vi "Gen - Remove Empty String Array.vi"(11 "Data Array":string[](array[string])) -> (3 "Data Out":string[](array[string]))   [LabVIEW 2020]
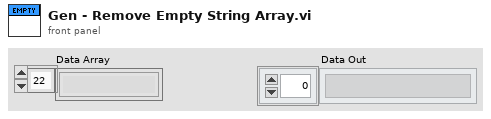
[diagram p1: front panel]
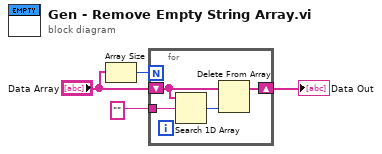
[diagram p0: block diagram]
diagram:
  n1 = Array Size(array="Data Array") -> (size(s)=w2:i32)
  n2 = for {
    N: w2 -> [_]
    tunnel: "" -> [w6]
    shift-right: [w7] -> w4
    shift-left: "Data Array" -> [w5]
    n3 = Search 1D Array(1D array=w5, element=w6) -> (index of element=w8:i32)  [unwired: 1 in]
    n4 = Delete From Array(array=w5, index=w8) -> (array with subset deleted=w7:string[])  [unwired: 1 in, 1 out]
  }
  "Data Out" <- w4
